vi "LarPeriscope.vi"(2 "Active?":bool, 9 "error in (no error)":errorcluster) -> (6 "error out":errorcluster)   [LabVIEW 2009]
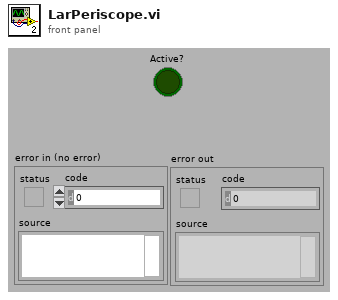
[diagram p1: front panel]
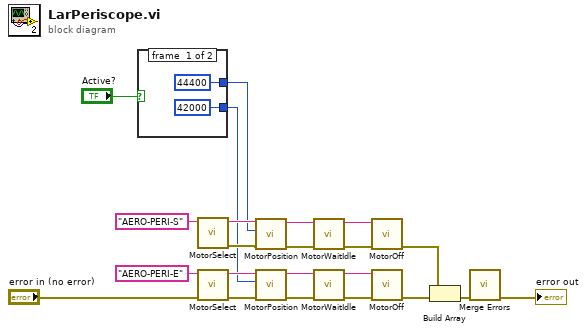
[diagram p0: block diagram]
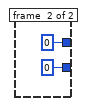
[diagram p2: hidden frame]
diagram:
  n1 = case shown="False" "Active?" {
    tunnel: [44400 ("Position") 0 ("Position")] -> w8
    tunnel: [42000 ("Position") 0 ("Position")] -> w7
    frame #0 {
    }
    frame #1 {
    }
  }
  n2 = call "MotorSelect.vi"("Motor"="AERO-PERI-S") -> ("Motor out"=w17:string, "error out"=w18:errorcluster)  [unwired: 7 in]
  n3 = call "MotorSelect.vi"("Motor"="AERO-PERI-E", "error in (no error)"="error in (no error)") -> ("Motor out"=w16:string, "error out"=w19:errorcluster)  [unwired: 6 in]
  n4 = call "MotorPosition.vi"("Motor"=w17, "Position"=w8, "error in (no error)"=w18) -> ("Motor out"=w14:string, "error out"=w15:errorcluster)  [unwired: 5 in]
  n5 = call "MotorPosition.vi"("Motor"=w16, "Position"=w7, "error in (no error)"=w19) -> ("Motor out"=w13:string, "error out"=w12:errorcluster)  [unwired: 5 in]
  n6 = call "MotorWaitIdle.vi"("Motor"=w14, "error in (no error)"=w15) -> ("Motor out"=w6:string, "error out"=w5:errorcluster)  [unwired: 6 in]
  n7 = call "MotorWaitIdle.vi"("Motor"=w13, "error in (no error)"=w12) -> ("Motor out"=w3:string, "error out"=w4:errorcluster)  [unwired: 6 in]
  n8 = call "MotorOff.vi"("Motor"=w6, "error in (no error)"=w5) -> ("error out"=w1:errorcluster)  [unwired: 6 in, 1 out]
  n9 = call "MotorOff.vi"("Motor"=w3, "error in (no error)"=w4) -> ("error out"=w2:errorcluster)  [unwired: 6 in, 1 out]
  n10 = Build Array(w1, w2) -> (w11:errorcluster[])
  n11 = call <vilib>:"Merge Errors.vi"("error array in"=w11) -> ("error out"=→"error out":errorcluster)  [unwired: 6 in]
